vi "OverlayBitmapTopLeft.vi"(7 "GroupName":string, 8 "error in":errorcluster, 9 "Bitmap":u32[][](array[colorbox]), 10 "TopLeft":T1, 11 "Image Reference In":T2) -> (0 "error out":errorcluster, 3 "Image Reference Out":T2)   [LabVIEW 2024, in "OpenLvVision_Overlays.lvlib"]
doc: "Overlays an bitmap on top of an image."
uses:
  OpenLvVision_Overlays.lvlib
  <vilib>/OpenLvVision/OpenLvVision_Image/Management/TypeDef/OLV Image.ctl
  TypeDefs/PointI32.ctl
  <vilib>/OpenLvVision/OpenLvVision_Image/Management/OLV Management.lvlib
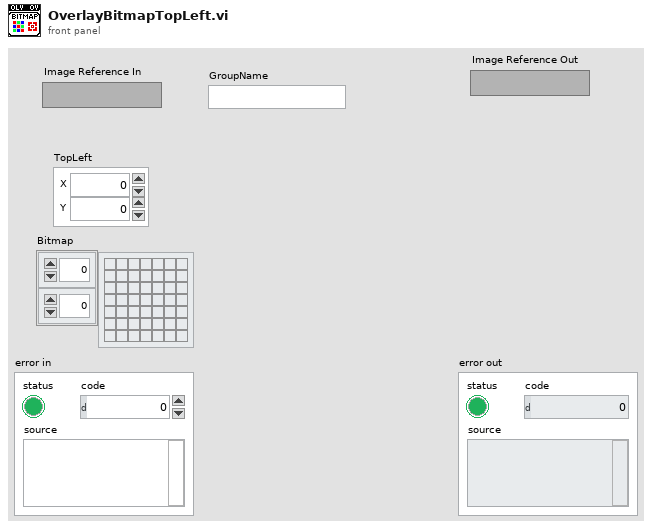
[diagram p1: front panel]
types:
  T1 = typedef "OpenLvVision_Overlays.lvlib/PointI32.ctl" = cluster{"X":i32, "Y":i32}
  T2 = typedef "OLV OpenLvVision_Image.lvlib/OLV Management.lvlib/OLV Image.ctl" = refnum<image>
  T3 = typedef "IMAQ Image.ctl" = refnum<image>
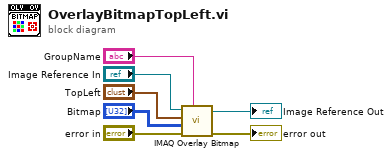
[diagram p0: block diagram]
diagram:
  n1 = call "IMAQ Overlay Bitmap"("Group"="GroupName", "error in (no error)"="error in", "Bitmap"="Bitmap", "Top Left Point"="TopLeft", "Image"="Image Reference In") -> ("error out"=→"error out":errorcluster, "Image Out"=→"Image Reference Out":T3)  [unwired: 5 in]
